vi "function B.vi"(0 "frequency 1":dbl, 1 "frequency 2":dbl, 2 "volume":dbl) -> (7 "Frequency Indicator":dbl, 8 "Frequency Indicator 2":dbl, 9 "Volume Indicator":dbl)   [LabVIEW 2016]
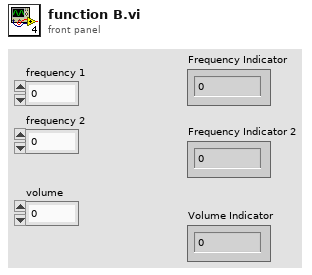
[diagram p1: front panel]
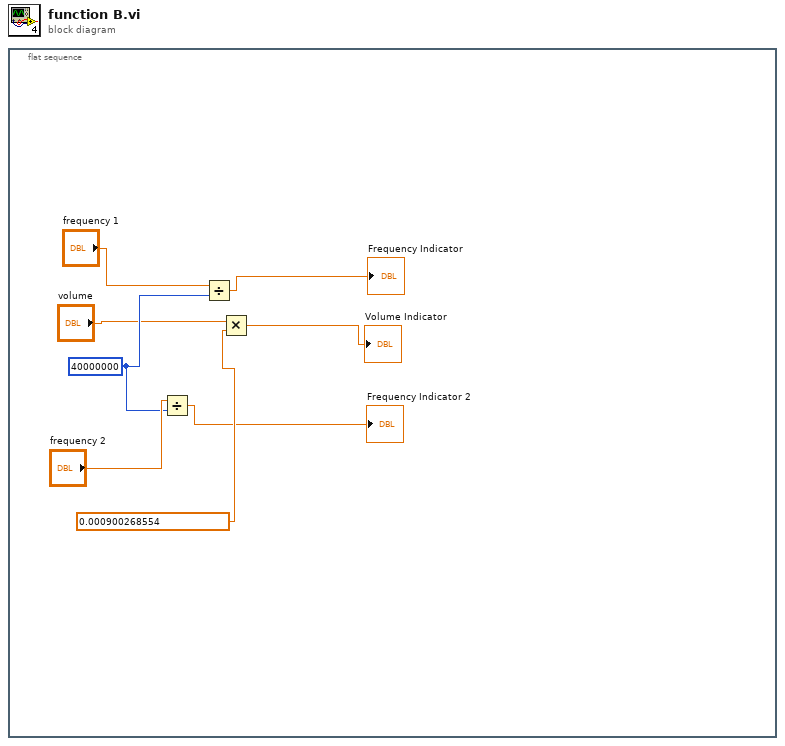
[diagram p0: block diagram]
diagram:
  n1 = flat-sequence {
    frame #0 {
      w5 = 40000000
      n2 = Divide(x="frequency 2", y=w5) -> (x/y=→"Frequency Indicator 2":dbl)
      n3 = Divide(x="frequency 1", y=w5) -> (x/y=→"Frequency Indicator":dbl)
      n4 = Multiply(x="volume", y=0.000900268554) -> (x*y=→"Volume Indicator":dbl)
    }
  }
